vi "Igor_EnsureIgorStringFormat.vi"(3 "Value":string) -> (1 "Value":string)   [LabVIEW 2019]
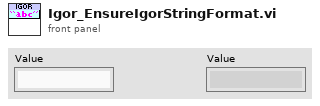
[diagram p1: front panel]
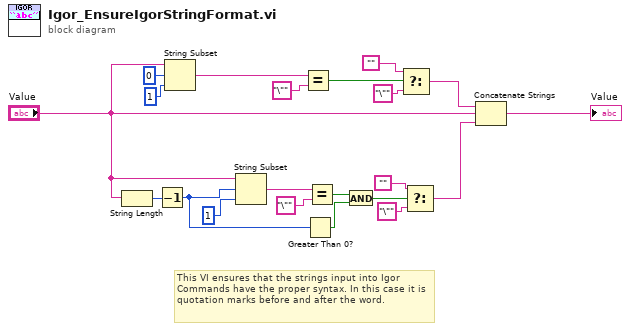
[diagram p0: block diagram]
diagram:
  # "This VI ensures that the strings input into Igor Commands have the proper syntax. In this case it is quotation marks before and after the word."
  n1 = String Length(string="Value") -> (length=w5:i32)
  n2 = Decrement(x=w5) -> (x-1=w4:i32)
  n3 = String Subset(string="Value", offset (0)=0, length (rest)=1 ("length (rest)")) -> (substring=w17:string)
  n4 = String Subset(string="Value", offset (0)=w4, length (rest)=1 ("length (rest)")) -> (substring=w12:string)
  n5 = Equal?(x=w17, y="\"") -> (x = y?=w18:bool)
  n6 = Greater Than 0?(x=w4) -> (x > 0?=w3:bool)
  n7 = Equal?(x=w12, y="\"") -> (x = y?=w2:bool)
  n8 = And(x=w2, y=w3) -> (x .and. y?=w1:bool)
  n9 = Select(t="" ("Empty String Constant"), s=w18, f="\"") -> (s? t:f=w11:string)
  n10 = Select(t="" ("Empty String Constant"), s=w1, f="\"") -> (s? t:f=w10:string)
  n11 = Concatenate Strings(w11, "Value", w10) -> (→"Value":string)
